vi "170519018sicaklikdegeridalgaformu.vi"() -> ()   [LabVIEW 2020]
panel:
  out "düsük":bool
  out "ayni":bool
  out "yüksek":bool
  in  "Sicaklik Degeri":u8
  out "DALGA FORMU":dbl(graph)
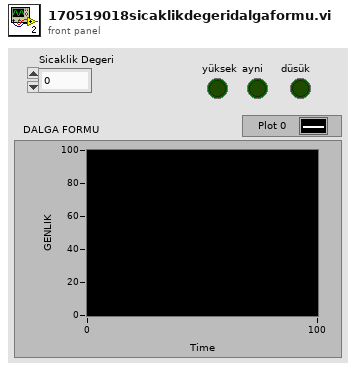
[diagram p1: front panel]
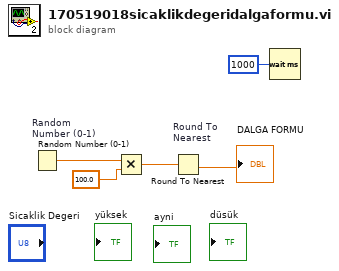
[diagram p0: block diagram]
diagram:
  n1 = Random Number (0-1) "Random \nNumber (0-1)"() -> (number: 0 to 1=w5:dbl)
  n2 = Multiply(x=w5, y=100.0) -> (x*y=w3:dbl)
  n3 = Round To Nearest "Round To \nNearest"(number=w3) -> (nearest integer value=→"DALGA FORMU":dbl)
  n4 = Wait (ms)(milliseconds to wait=u32 1000) -> ()  [unwired: 1 out]
